vi "Create UUT Instances and Aliases.vi"(8 "error in":errorcluster) -> (0 "error out":errorcluster, 4 "log":string)   [LabVIEW 2024]
uses:
  <vilib>/Plug-In SDKs/Clients/Metadata/UUT Instance.ctl
  <vilib>/Plug-In SDKs/Clients/Metadata/Extension.ctl
  <vilib>/Plug-In SDKs/Clients/Metadata Store V1/Metadata Store Client.lvlibp/API/Metadata Store V1/Create UUT Instance.vi
  <vilib>/Plug-In SDKs/Clients/Metadata Store V1/Metadata Store Client.lvlibp/API/Metadata Store V1/Create Alias (Metadata - UUT Instance).vi
  <vilib>/Plug-In SDKs/Clients/Metadata Store V1/Metadata Store Client.lvlibp
  <vilib>/Plug-In SDKs/Clients/Metadata/NI Metadata Types.lvlib
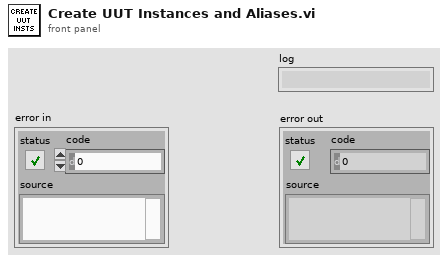
[diagram p1: front panel]
types:
  T1 = typedef "NI Metadata Types.lvlib/UUT Instance.ctl" = cluster{"serial number":string, "manufacture date":string, "firmware version":string, "hardware version":string, "id":string, "uut id":string, "link":string, "extension":T2[], "schema id":string}
  T2 = typedef "NI Metadata Types.lvlib/Extension.ctl" = cluster{"name":string, "value":string}
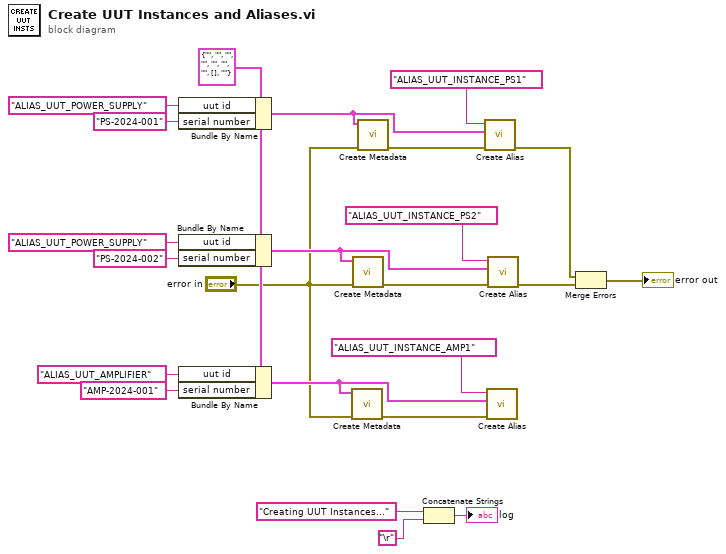
[diagram p0: block diagram]
diagram:
  w5 = T1 {"serial number"="", "manufacture date"="", "firmware version"="", "hardware version"="", "id"="", "uut id"="", "link"="", "extension"=[], "schema id"=""} ("uut instance")
  n1 = Bundle By Name(cluster=w5, "uut id"="ALIAS_UUT_POWER_SUPPLY" ("operator name"), "serial number"="PS-2024-001" ("operator name")) -> (w17:T1)
  n2 = Bundle By Name(cluster=w5, "uut id"="ALIAS_UUT_POWER_SUPPLY" ("serial number"), "serial number"="PS-2024-002" ("model")) -> (w20:T1)
  n3 = Bundle By Name(cluster=w5, "uut id"="ALIAS_UUT_AMPLIFIER" ("serial number"), "serial number"="AMP-2024-001" ("model")) -> (w6:T1)
  n4 = call-poly <vilib>:"Create Metadata.vi"("error in"="error in", "uut instance"=w6) -> ("error out"=w8:errorcluster)  [unwired: 8 in, 1 out]
  n5 = call-poly <vilib>:"Create Metadata.vi"("error in"="error in", "uut instance"=w20) -> ("error out"=w15:errorcluster)  [unwired: 8 in, 1 out]
  n6 = call-poly <vilib>:"Create Metadata.vi"("error in"="error in", "uut instance"=w17) -> ("error out"=w16:errorcluster)  [unwired: 8 in, 1 out]
  n7 = Concatenate Strings("Creating UUT Instances..." ("role"), "\r") -> (→"log":string)
  n8 = call-poly <vilib>:"Create Alias.vi"("error in"=w16, "uut instance"=w17, "alias name"="ALIAS_UUT_INSTANCE_PS1") -> ("error out"=w21:errorcluster)  [unwired: 7 in, 1 out]
  n9 = call-poly <vilib>:"Create Alias.vi"("error in"=w8, "uut instance"=w6, "alias name"="ALIAS_UUT_INSTANCE_AMP1") -> ()  [unwired: 7 in, 2 out]
  n10 = call-poly <vilib>:"Create Alias.vi"("error in"=w15, "uut instance"=w20, "alias name"="ALIAS_UUT_INSTANCE_PS2") -> ("error out"=w22:errorcluster)  [unwired: 7 in, 1 out]
  n11 = Merge Errors(w21, w22) -> (→"error out":errorcluster)
